vi "sectors checker.vi"(8 "error in (no error)":errorcluster, 10 "array2":string[][](array[string]), 11 "array1":string[][](array[string])) -> (0 "error out":errorcluster)   [LabVIEW 2024]
uses:
  443d4004-14de-444d-9e4b-623f00349db9.vi
  <vilib>/Utility/error.llb/Error Cluster From Error Code.vi
  <vilib>/ErrorRing/Error Ring.xnode
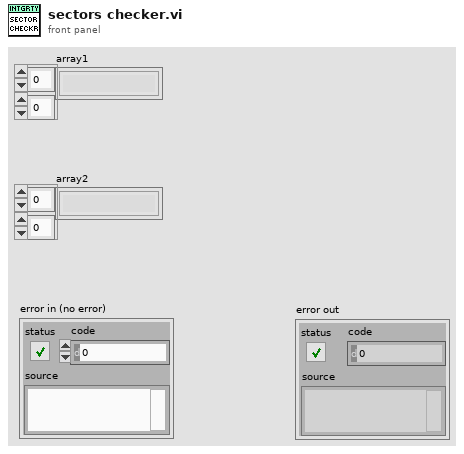
[diagram p1: front panel]
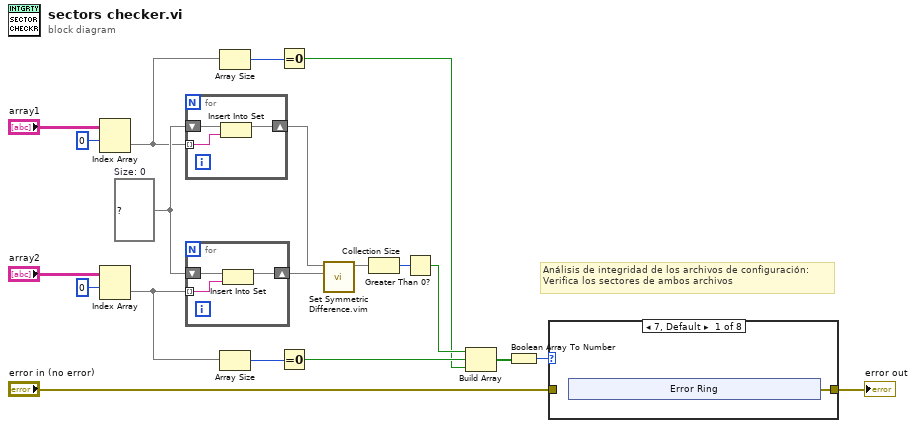
[diagram p0: block diagram]
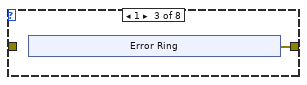
[diagram p3: hidden frame]
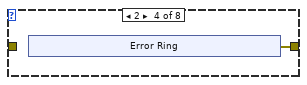
[diagram p4: hidden frame]
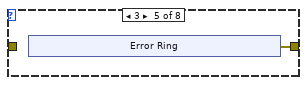
[diagram p5: hidden frame]
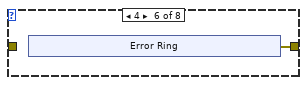
[diagram p6: hidden frame]
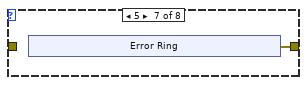
[diagram p7: hidden frame]
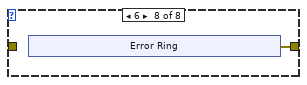
[diagram p8: hidden frame]
diagram:
  w17 = set{string} {}  # Size: 0
  # "Análisis de integridad de los archivos de configuración:\nVerifica los sectores de ambos archivos"
  n1 = Index Array(array="array1", index (row)=0) -> (element=w10:string[])  [unwired: 1 in]
  n2 = Index Array(array="array2", index (row)=0) -> (element=w8:string[])  [unwired: 1 in]
  n3 = for {
    shift-right: [w22] -> w16
    shift-left: w17 -> [w23]
    tunnel: w10 -> [w21] mode=indexing
    n4 = Insert Into Set(10:w21, 11:w23) -> (3:w22:set{string})  [unwired: 1 out]
  }
  n5 = for {
    shift-right: [w25] -> w15
    shift-left: w17 -> [w26]
    tunnel: w8 -> [w24] mode=indexing
    n6 = Insert Into Set(10:w24, 11:w26) -> (3:w25:set{string})  [unwired: 1 out]
  }
  n7 = Array Size(array=w10) -> (size(s)=w11:i32)
  n8 = Array Size(array=w8) -> (size(s)=w9:i32)
  n9 = Equal To 0?(x=w11) -> (x = 0?=w1:bool)
  n10 = Equal To 0?(x=w9) -> (x = 0?=w7:bool)
  n11 = call "Set Symmetric Difference.vim"("set 2"=w15, "set 1"=w16) -> ("symmetric difference"=w14:set{string})  [unwired: 9 in]
  n12 = Collection Size(1:w14) -> (0:w13:i32)
  n13 = Greater Than 0?(x=w13) -> (x > 0?=w2:bool)
  n14 = Build Array(w2, w7, w1) -> (w6:bool[])
  n15 = Boolean Array To Number(Boolean array=w6) -> (number=w5:u32)
  n16 = case shown="7, Default" w5 {
    tunnel: "error in (no error)" -> [_ w33 _ _ _ _ _ _]
    tunnel: [w27 w33 w34 w40 w46 w52 w58 w64] -> w3
    frame 7, Default {
      n17 = xnode "Error Ring"() -> ("error out"=w27:errorcluster)
    }
    frame 0 {
    }
    frame 1 {
      n18 = xnode "Error Ring"() -> ("error out"=w34:errorcluster)
    }
    frame 2 {
      n19 = xnode "Error Ring"() -> ("error out"=w40:errorcluster)
    }
    frame 3 {
      n20 = xnode "Error Ring"() -> ("error out"=w46:errorcluster)
    }
    frame 4 {
      n21 = xnode "Error Ring"() -> ("error out"=w52:errorcluster)
    }
    frame 5 {
      n22 = xnode "Error Ring"() -> ("error out"=w58:errorcluster)
    }
    frame 6 {
      n23 = xnode "Error Ring"() -> ("error out"=w64:errorcluster)
    }
  }
  "error out" <- w3
